vi "Excel_CloseReference_v2.vi"(7 "Keep Excel Open ?":bool, 8 "error in (no error)":errorcluster, 9 "Sheets Reference In":refnum<k7>, 10 "Workbook Reference In":refnum<k7>, 11 "Excel Application Reference In":refnum<k7>) -> (0 "error out":errorcluster, 3 "Excel Application Reference Out":refnum<k7>)   [LabVIEW 2014]
doc: "This VI demonstrates the use of ActiveX to write a table into a Microsoft Excel worksheet."
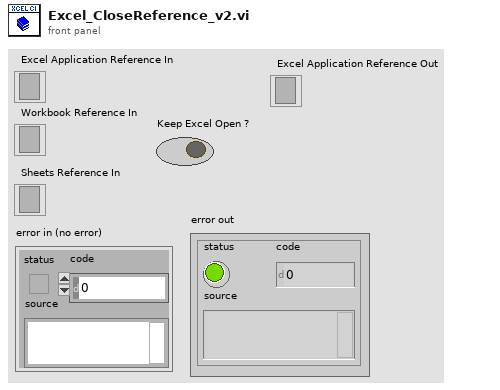
[diagram p1: front panel]
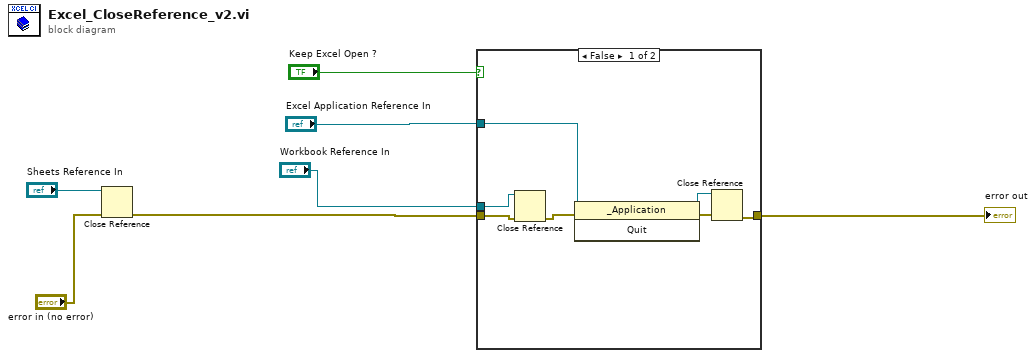
[diagram p0: block diagram]
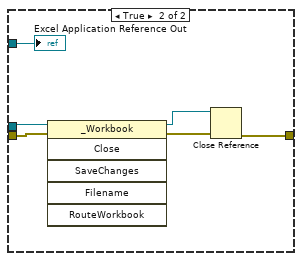
[diagram p2: hidden frame]
diagram:
  n1 = Close Reference(reference="Sheets Reference In", error in (no error)="error in (no error)") -> (error out=w5:errorcluster)
  n2 = case shown="False" "Keep Excel Open ?" {
    tunnel: w5 -> [w14 w17]
    tunnel: "Workbook Reference In" -> [w13 w18]
    tunnel: [w8 w20] -> w3
    tunnel: "Excel Application Reference In" -> [w11 w19]
    frame False {
      n3 = Close Reference(reference=w13, error in (no error)=w14) -> (error out=w12:errorcluster)
      n4 = invoke class="_Application" method="Quit"(reference=w11, error in=w12) -> (reference out=w9:refnum<k7>, error out=w10:errorcluster)  [unwired: 1 in, 1 out]
      n5 = Close Reference(reference=w9, error in (no error)=w10) -> (error out=w8:errorcluster)
    }
    frame True {
      n6 = invoke class="_Workbook" method="Close"(reference=w18, error in=w17) -> (reference out=w15:refnum<k7>, error out=w16:errorcluster)  [unwired: 4 in, 4 out]
      n7 = Close Reference(reference=w15, error in (no error)=w16) -> (error out=w20:errorcluster)
      "Excel Application Reference Out" <- w19
    }
  }
  "error out" <- w3
